vi "Numeric Output Item Resize.vi"(8 "error in (no error)":errorcluster, 9 "NewBnds":T2, 10 "Numeric UI Elements":T1, 11 "Output":T3) -> (0 "error out":errorcluster)   [LabVIEW 2015, in "OutputUI.lvclass"]
uses:
  OutputUI.lvclass
  Step/STEP_OUTPUT.ctl
  Step/OUTPUT_DATA_TYPE.ctl
  OUTPUT_CHECK_TYPE.ctl
  Step/OUTPUT_VALUE_TYPE.ctl
  <vilib>/Utility/miscctls.llb/LVRectTypeDef.ctl
  Step.lvclass
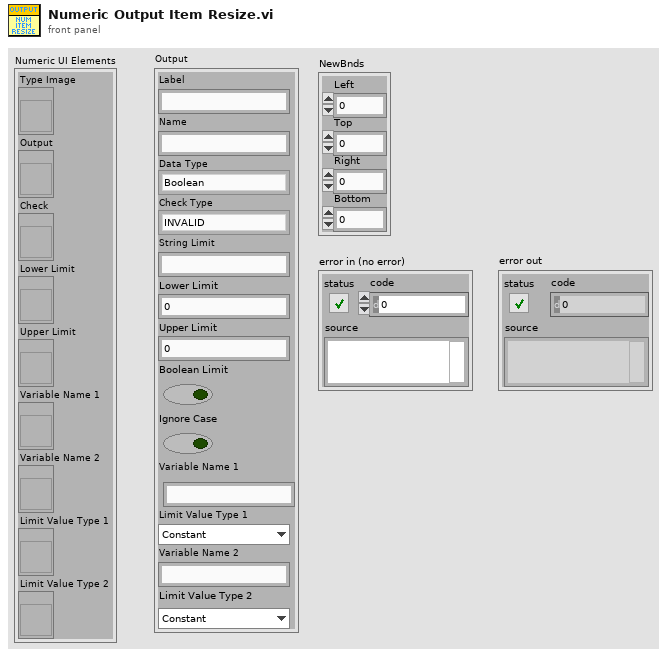
[diagram p1: front panel]
types:
  T1 = cluster{"Type Image":refnum<vi>, "Output":refnum<vi>, "Check":refnum<vi>, "Lower Limit":refnum<vi>, "Upper Limit":refnum<vi>, "Variable Name 1":refnum<vi>, "Variable Name 2":refnum<vi>, "Limit Value Type 1":refnum<vi>, "Limit Value Type 2":refnum<vi>}
  T2 = typedef "LVRectTypeDef.ctl" = cluster{"Left":i16, "Top":i16, "Right":i16, "Bottom":i16}
  T3 = typedef "Step.lvclass/STEP_OUTPUT.ctl" = cluster{"Label":string, "Name":string, "Data Type":T4, "Check Type":T5, "String Limit":string, "Lower Limit":dbl, "Upper Limit":dbl, "Boolean Limit":bool, "Ignore Case":bool, "Variable Name 1":string, "Limit Value Type 1":T6, "Variable Name 2":string, "Limit Value Type 2":T6}
  T4 = typedef "Step.lvclass/OUTPUT_DATA_TYPE.ctl" = enum16{"Boolean", "String", "Numeric", "Other"}
  T5 = typedef "Step.lvclass/OUTPUT_CHECK_TYPE.ctl" = enum16{"INVALID", "DO_NOT_CHECK", "RECORD", "VARIABLE", "EQUAL", "NOT_EQUAL", "STR_CONTAINS", "STR_START_WITH", "STR_END_WITH", "STR_REGEX_MATCH", "NUM_GT", "NUM_LT", "NUM_GE", "NUM_LE", "NUM_RANGE", "NUM_RANGE_BDY"}
  T6 = typedef "Step.lvclass/OUTPUT_VALUE_TYPE.ctl" = enum16{"Constant", "Variable"}
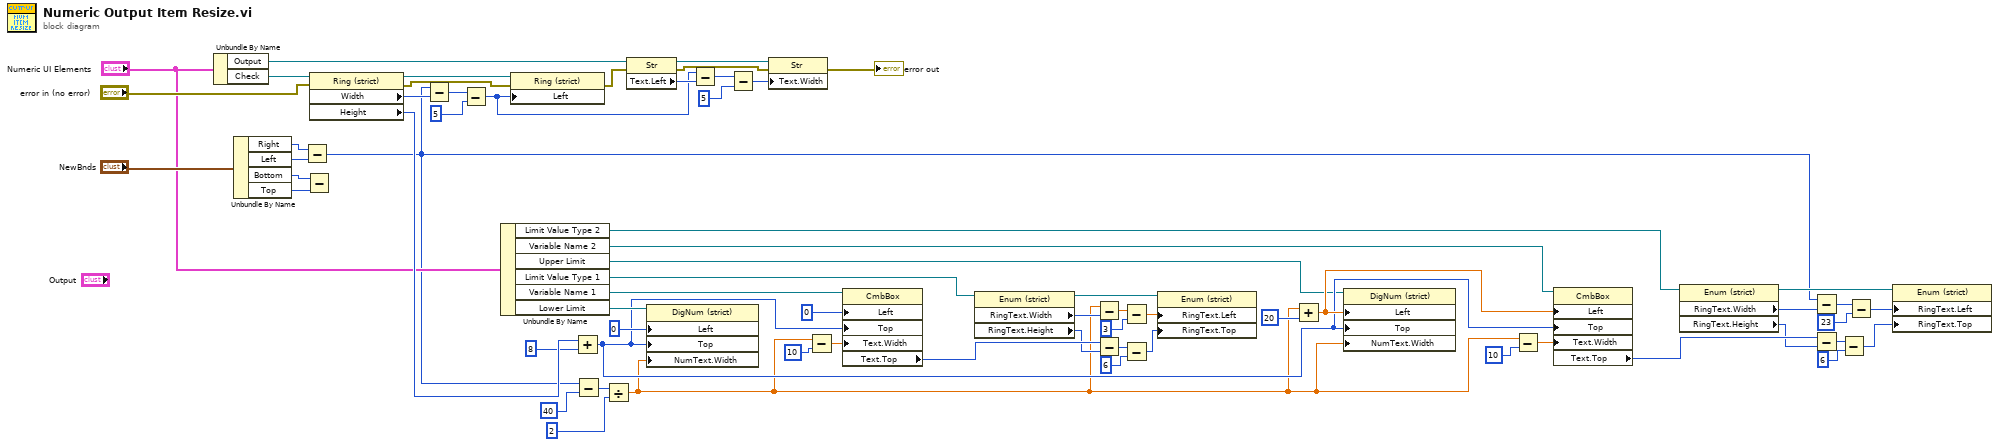
[diagram p0: block diagram]
diagram:
  n1 = Unbundle By Name("Numeric UI Elements") -> ("Output"=w57:refnum<vi>, "Check"=w65:refnum<vi>)
  n2 = Unbundle By Name("NewBnds") -> ("Right"=w62:i16, "Left"=w63:i16, "Bottom"=w61:i16, "Top"=w60:i16)
  n3 = Subtract(x=w62, y=w63) -> (x-y=w7:i16)
  n4 = Subtract(x=w61, y=w60) -> ()  [unwired: 1 out]
  n5 = property class="Ring (strict)"(reference=w65, error in="error in (no error)") -> (reference out=w59:refnum<vi>, error out=w46:errorcluster, "Width"=w58:u32, "Height"=w43:u32)
  n6 = Subtract(x=w7, y=w58) -> (x-y=w54:u32)
  n7 = Subtract(x=w54, y=5) -> (x-y=w52:u32)
  n8 = Unbundle By Name("Numeric UI Elements") -> ("Limit Value Type 2"=w17:refnum<vi>, "Variable Name 2"=w32:refnum<vi>, "Upper Limit"=w29:refnum<vi>, "Limit Value Type 1"=w24:refnum<vi>, "Variable Name 1"=w34:refnum<vi>, "Lower Limit"=w41:refnum<vi>)
  n9 = property class="Ring (strict)"(reference=w59, error in=w46, "Left"=w52) -> (error out=w45:errorcluster)  [unwired: 1 out]
  n10 = Add(x=w43, y=8) -> (x+y=w30:u32)
  n11 = Subtract(x=w7, y=i16 40) -> (x-y=w37:i16)
  n12 = Divide(x=w37, y=i16 2) -> (x/y=w13:dbl)
  n13 = property class="Str"(reference=w57, error in=w45) -> (reference out=w56:refnum<vi>, error out=w44:errorcluster, "Text.Left"=w55:i32)
  n14 = property class="DigNum (strict)"(reference=w41, "Left"=0 ("Position:Left"), "Top"=w30, "NumText.Width"=w13) -> ()  [unwired: 1 in, 2 out]
  n15 = Subtract(x=w52, y=w55) -> (x-y=w51:u32)
  n16 = Subtract(x=w51, y=u32 5) -> (x-y=w50:u32)
  n17 = property class="Str"(reference=w56, error in=w44, "Text.Width"=w50) -> (error out=→"error out":errorcluster)  [unwired: 1 out]
  n18 = Subtract(x=w13, y=10) -> (x-y=w27:dbl)
  n19 = property class="CmbBox"(reference=w34, "Left"=0, "Top"=w30, "Text.Width"=w27) -> ("Text.Top"=w22:i32)  [unwired: 1 in, 2 out]
  n20 = property class="Enum (strict)"(reference=w24) -> (reference out=w23:refnum<vi>, "RingText.Width"=w15:u32, "RingText.Height"=w21:u32)  [unwired: 1 in, 1 out]
  n21 = Subtract(x=w13, y=w15) -> (x-y=w3:dbl)
  n22 = Subtract(x=w22, y=w21) -> (x-y=w20:u32)
  n23 = Subtract(x=w3, y=3) -> (x-y=w2:dbl)
  n24 = Subtract(x=w20, y=u32 6) -> (x-y=w18:u32)
  n25 = property class="Enum (strict)"(reference=w23, "RingText.Left"=w2, "RingText.Top"=w18) -> ()  [unwired: 1 in, 2 out]
  n26 = Add(x=w13, y=20) -> (x+y=w31:dbl)
  n27 = property class="DigNum (strict)"(reference=w29, "Left"=w31, "Top"=w30, "NumText.Width"=w13) -> ()  [unwired: 1 in, 2 out]
  n28 = Subtract(x=w13, y=10) -> (x-y=w25:dbl)
  n29 = property class="CmbBox"(reference=w32, "Left"=w31, "Top"=w30, "Text.Width"=w25) -> ("Text.Top"=w10:i32)  [unwired: 1 in, 2 out]
  n30 = property class="Enum (strict)"(reference=w17) -> (reference out=w16:refnum<vi>, "RingText.Width"=w14:u32, "RingText.Height"=w9:u32)  [unwired: 1 in, 1 out]
  n31 = Subtract(x=w7, y=w14) -> (x-y=w6:u32)
  n32 = Subtract(x=w10, y=w9) -> (x-y=w11:u32)
  n33 = Subtract(x=w11, y=u32 6) -> (x-y=w8:u32)
  n34 = Subtract(x=w6, y=u32 23) -> (x-y=w4:u32)
  n35 = property class="Enum (strict)"(reference=w16, "RingText.Left"=w4, "RingText.Top"=w8) -> ()  [unwired: 1 in, 2 out]
